vi "OutputToXML.vi"(8 "error in (no error)":errorcluster, 11 "RingdownPlugin in":refnum<class "RingdownPlugin.lvclass">) -> (0 "error out":errorcluster, 2 "AppOutputData out":variant)   [LabVIEW 2014, in "AppPlugins.lvlib" / "RingdownPlugin.lvclass"]
uses:
  RingdownPlugin.lvclass
  TypeDef/RingdownOutput.ctl
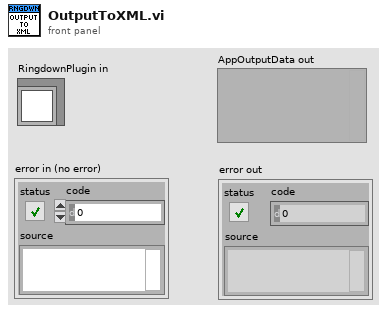
[diagram p1: front panel]
types:
  T1 = typedef "AppPlugins.lvlib/RingdownPlugin.lvclass/RingdownOutput.ctl" = cluster{"FramesPerSecond":dbl, "PronyEstimate":dbl[], "RingdownParameters":cluster{"Amplitude":dbl[], "Damping":dbl[], "Frequency":dbl[], "Phase":dbl[]}, "ReportingTime":dbl, "DataSize":u32, "InputSignal":dbl[]}
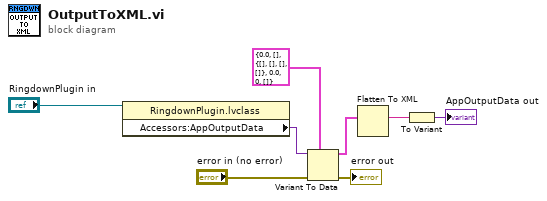
[diagram p0: block diagram]
diagram:
  n1 = property class="RingdownPlugin.lvclass"(reference="RingdownPlugin in") -> ("Accessors:AppOutputData"=w6:variant)  [unwired: 1 in, 2 out]
  n2 = Variant To Data(error in="error in (no error)", type=T1 {"FramesPerSecond"=0.0, "PronyEstimate"=[], "RingdownParameters"={"Amplitude"=[], "Damping"=[], "Frequency"=[], "Phase"=[]}, "ReportingTime"=0.0, "DataSize"=0, "InputSignal"=[]} ("RingdownOutput"), Variant=w6) -> (data=w5:T1, error out=→"error out":errorcluster)
  n3 = Flatten To XML(anything=w5) -> (xml string=w4:string)
  n4 = To Variant(anything=w4) -> (Variant=→"AppOutputData out":variant)
